vi "SLL DE AO Response LV2Global.vi"(6 "Option":T1=enum."Send Response", 8 "Error in (no error)":errorcluster, 11 "Executed For?":string) -> (0 "Error out":errorcluster, 3 "Found?":bool)   [LabVIEW 2013]
uses:
  Controls/SLL DE AO Response LV2Global Options.ctl
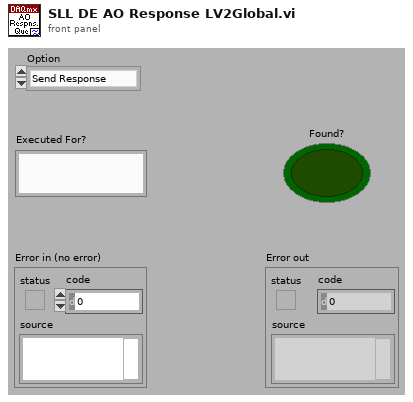
[diagram p1: front panel]
types:
  T1 = typedef "SLL DE AO Response LV2Global Options.ctl" = enum16{"Initialize", "Send Response", "Check Response", "Close"}
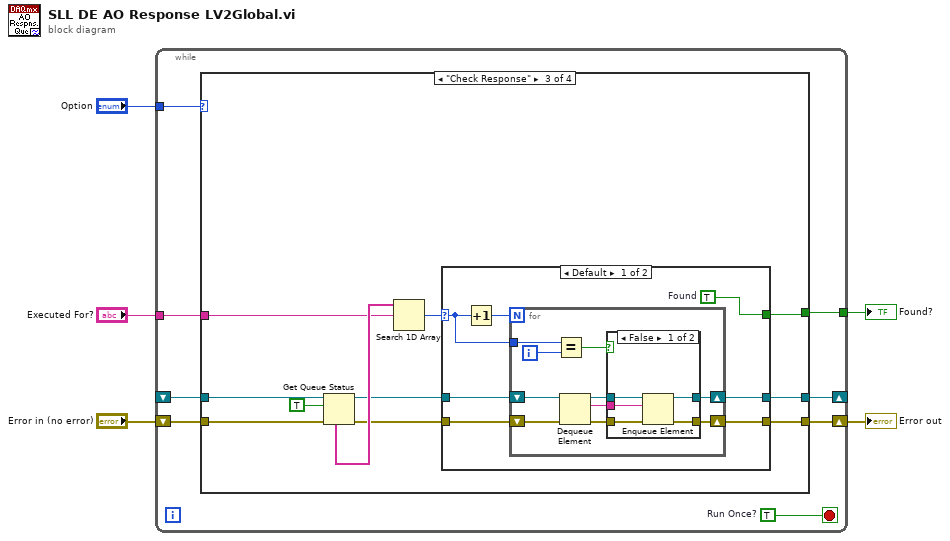
[diagram p0: block diagram]
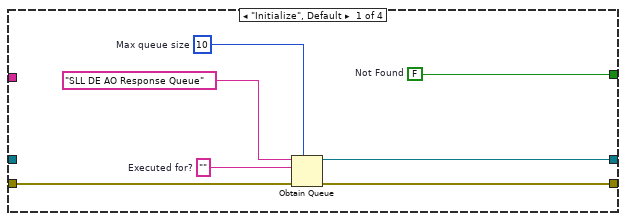
[diagram p2: hidden frame]
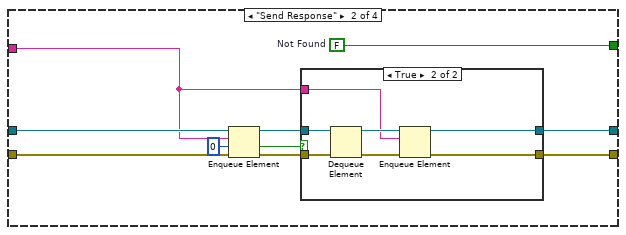
[diagram p3: hidden frame]
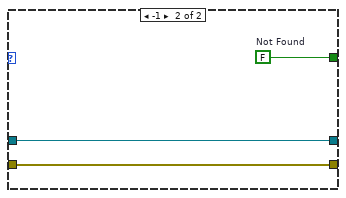
[diagram p6: hidden frame]
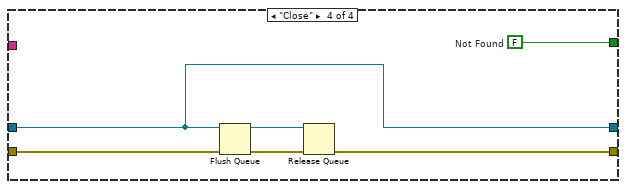
[diagram p7: hidden frame]
diagram:
  n1 = while {
    tunnel: "Option" -> [w12]
    shift-right: [w11] -> _
    shift-left: _ -> [w10]
    tunnel: "Executed For?" -> [w9]
    shift-right: [w7] -> w2
    shift-left: "Error in (no error)" -> [w8]
    tunnel: [w6] -> w1
    stop <- w13 stop-if-true
    w13 = TRUE  # Run Once?
    n2 = case shown="\"Check Response\"" w12 {
      tunnel: [w16 w22 w40 w78] -> w11
      tunnel: w10 -> [_ w28 w47 w78]
      tunnel: w9 -> [_ w21 w44 _]
      tunnel: w8 -> [w18 w27 w48 w79]
      tunnel: [w17 w23 w39 w77] -> w7
      tunnel: [w14 w26 w38 w76] -> w6
      frame "Initialize", Default {
        w14 = FALSE  # Not Found
        w15 = 10  # Max queue size
        w19 = ""  # Executed for?
        n3 = Obtain Queue(max queue size (-1, unlimited)=w15, name (unnamed)="SLL DE AO Response Queue", element data type=w19, error in (no error)=w18) -> (queue out=w16:refnum<queue>, error out=w17:errorcluster)  [unwired: 1 in, 1 out]
      }
      frame "Send Response" {
        w26 = FALSE  # Not Found
        n4 = Enqueue Element(queue=w28, element=w21, timeout in ms (-1)=0, error in (no error)=w27) -> (queue out=w22:refnum<queue>, timed out?=w24:bool, error out=w23:errorcluster)
        n5 = case shown="True" w24 {
          tunnel: w23 -> [w30 w36]
          tunnel: w22 -> [w29 w37]
          tunnel: [w30 w34] -> _
          tunnel: [w29 w33] -> _
          tunnel: w21 -> [_ w31]
          frame False {
          }
          frame True {
            n6 = Dequeue Element(queue=w37, error in (no error)=w36) -> (queue out=w32:refnum<queue>, error out=w35:errorcluster)  [unwired: 1 in, 2 out]
            n7 = Enqueue Element(queue=w32, element=w31, error in (no error)=w35) -> (queue out=w33:refnum<queue>, error out=w34:errorcluster)  [unwired: 1 in, 1 out]
          }
        }
      }
      frame "Check Response" {
        n8 = Get Queue Status(queue=w47, return elements? (F)=TRUE, error in (no error)=w48) -> (queue out=w42:refnum<queue>, error out=w41:errorcluster, elements=w45:string[])  [unwired: 5 out]
        n9 = Search 1D Array(1D array=w45, element=w44) -> (index of element=w43:i32)  [unwired: 1 in]
        n10 = case shown="Default" w43 {
          selector: w43 -> [w49 _]
          tunnel: w42 -> [w52 w75]
          tunnel: w41 -> [w55 w74]
          tunnel: [w54 w75] -> w40
          tunnel: [w53 w74] -> w39
          tunnel: [w51 w73] -> w38
          frame Default {
            w51 = TRUE  # Found
            n11 = Increment(x=w49) -> (x+1=w50:i32)
            n12 = for {
              N: w50 -> [_]
              shift-right: [w61] -> w54
              shift-left: w52 -> [w64]
              shift-right: [w60] -> w53
              shift-left: w55 -> [w65]
              tunnel: w49 -> [w58]
              i -> [w57]
              n13 = Equal?(x=w58, y=w57) -> (x = y?=w56:bool)
              n14 = Dequeue Element(queue=w64, error in (no error)=w65) -> (queue out=w63:refnum<queue>, element=w59:string, error out=w62:errorcluster)  [unwired: 1 in, 1 out]
              n15 = case shown="False" w56 {
                tunnel: w63 -> [w70 w72]
                tunnel: w62 -> [w68 w71]
                tunnel: [w69 w72] -> w61
                tunnel: [w67 w71] -> w60
                tunnel: w59 -> [w66 _]
                frame False {
                  n16 = Enqueue Element(queue=w70, element=w66, error in (no error)=w68) -> (queue out=w69:refnum<queue>, error out=w67:errorcluster)  [unwired: 1 in, 1 out]
                }
                frame True {
                }
              }
            }
          }
          frame -1 {
            w73 = FALSE  # Not Found
          }
        }
      }
      frame "Close" {
        w76 = FALSE  # Not Found
        n17 = Flush Queue(queue=w78, error in (no error)=w79) -> (queue out=w81:refnum<queue>, error out=w80:errorcluster)  [unwired: 1 out]
        n18 = Release Queue(queue=w81, error in (no error)=w80) -> (error out=w77:errorcluster)  [unwired: 1 in, 2 out]
      }
    }
  }
  "Error out" <- w2
  "Found?" <- w1
